vi "WaitForRPM.vi"(7 "Notifier Data":T2, 8 "error in (no error)":errorcluster, 9 "RPM target":dbl, 10 "Data Cluster":T1, 11 "Notifier in":refnum<notifier>) -> (0 "error out":errorcluster, 1 "RPM Target Reached":bool, 2 "STOP Button Pressed":bool, 3 "RPM Timeout":bool, 5 "RPM":dbl)   [LabVIEW 2026, in "Acquisition.lvlib"]
uses:
  Acquisition.lvlib
  controls/NotifierAndDataQueue.ctl
  controls/WaveformChartData.ctl
  Hardware Configuration.ctl
  Settings/Settings.lvlib
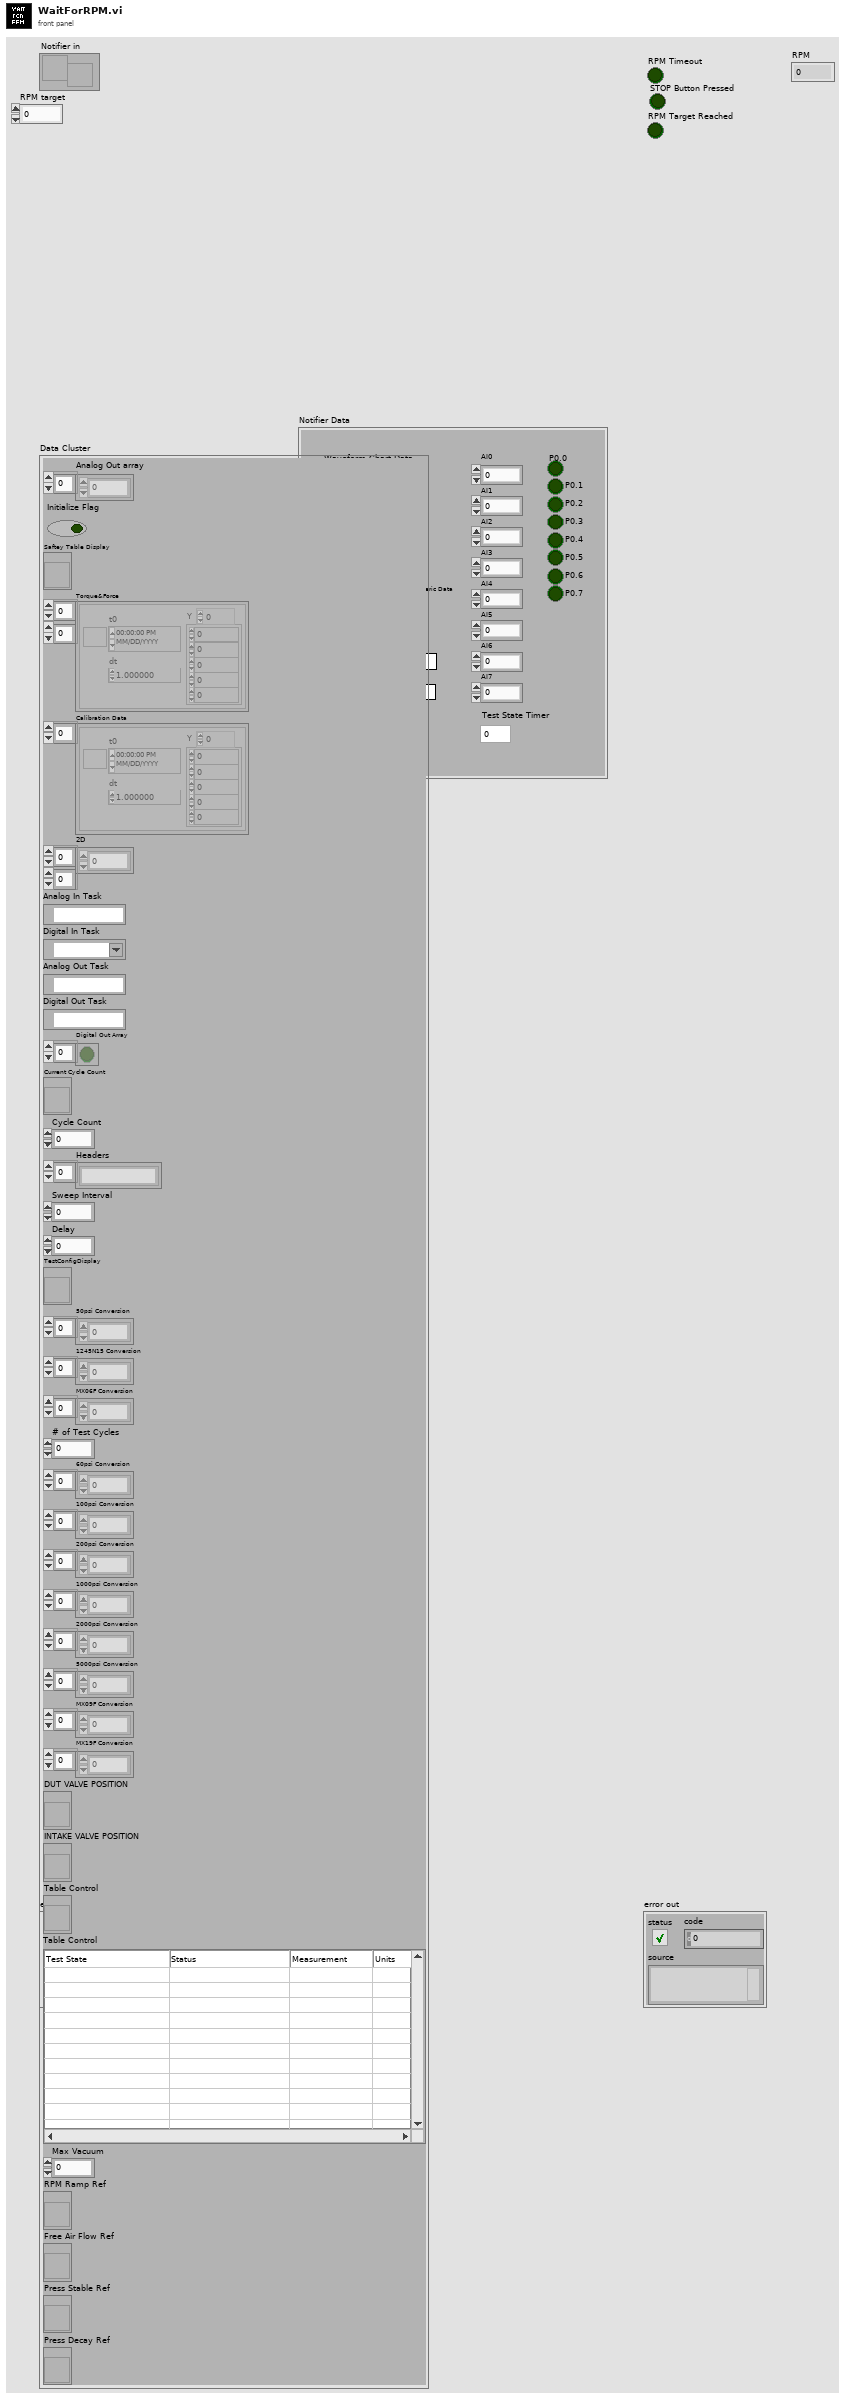
[diagram p1: front panel]
types:
  T1 = typedef "Acquisition.lvlib/Hardware Configuration.ctl" = cluster{"Analog Out array":dbl[], "Initialize Flag":bool, "Saftey Table Display":refnum<vi>, "Torque&Force":waveform(dbl)[][], "Calibration Data":waveform(dbl)[], "2D":dbl[][], "Analog In Task":refnum<k21>, "Digital In Task":refnum<k21>, "Analog Out Task":refnum<k21>, "Digital Out Task":refnum<k21>, "Digital Out Array":bool[], "Current Cycle Count":refnum<vi>, "Cycle Count":u64, "Headers":string[], "Sweep Interval":u64, "Delay":u64, "TestConfigDisplay":refnum<vi>, "50psi Conversion":dbl[], "1245N15 Conversion":dbl[], "MX06F Conversion":dbl[], "# of Test Cycles":u64, "60psi Conversion":dbl[], "100psi Conversion":dbl[], "200psi Conversion":dbl[], "1000psi Conversion":dbl[], "2000psi Conversion":dbl[], "5000psi Conversion":dbl[], "MX09F Conversion":dbl[], "MX19F Conversion":dbl[], "DUT VALVE POSITION":refnum<vi>, "INTAKE VALVE POSITION":refnum<vi>, "Table Control":refnum<vi>, "Table Control":string[][], "Max Vacuum":dbl, "RPM Ramp Ref":refnum<vi>, "Free Air Flow Ref":refnum<vi>, "Press Stable Ref":refnum<vi>, "Press Decay Ref":refnum<vi>}
  T2 = typedef "NotifierAndDataQueue.ctl" = cluster{"Ai0":dbl, "Ai1":dbl, "Ai2":dbl, "Ai3":dbl, "Ai4":dbl, "Ai5":dbl, "Ai6":dbl, "Ai7":dbl, "P0.0":bool, "P0.1":bool, "P0.2":bool, "P0.3":bool, "P0.4":bool, "P0.5":bool, "P0.6":bool, "P0.7":bool, "2D Numeric Data":dbl[][], "String 2":string, "String 1":string, "Waveform Chart Data":T3, "Test State Timer":dbl}
  T3 = typedef "Settings.lvlib/WaveformChartData.ctl" = cluster{"DUT Vacuum":dbl, "Motor RPM":dbl, "DUT RPM":dbl, "Tank Vacuum":dbl}
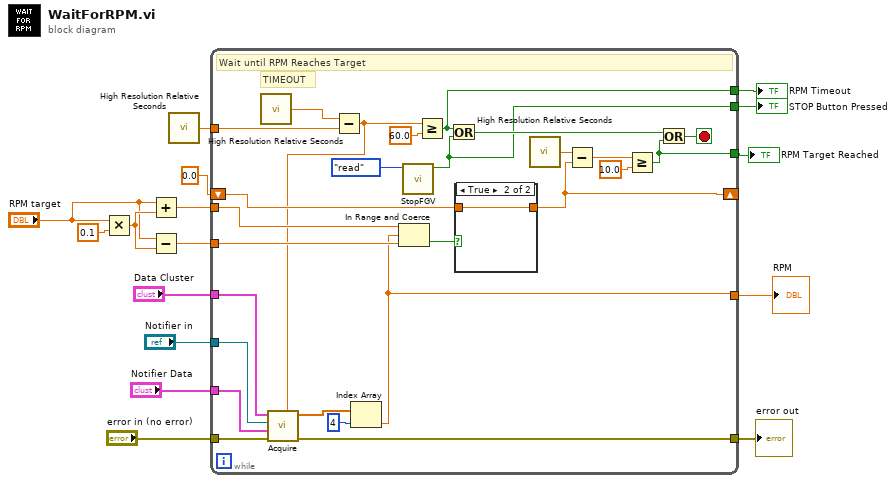
[diagram p0: block diagram]
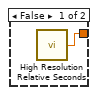
[diagram p2: hidden frame]
diagram:
  n1 = Multiply(x="RPM target", y=0.1) -> (x*y=w8:dbl)
  n2 = Add(x="RPM target", y=w8) -> (x+y=w7:dbl)
  n3 = Subtract(x="RPM target", y=w8) -> (x-y=w6:dbl)
  n4 = call <vilib>:"High Resolution Relative Seconds.vi"() -> ("relative seconds"=w16:dbl)
  n5 = while {
    tunnel: "Notifier in" -> [w40]
    tunnel: "error in (no error)" -> [w42]
    tunnel: [w41] -> w11
    tunnel: "Notifier Data" -> [w37]
    tunnel: "Data Cluster" -> [w36]
    tunnel: w7 -> [w33]
    tunnel: w6 -> [w32]
    shift-right: [w29] -> _
    shift-left: 0.0 ("relative seconds") -> [w28]
    tunnel: w16 -> [w24]
    tunnel: [w21] -> w4
    tunnel: [w20] -> w3
    tunnel: [w19] -> w2
    tunnel: [w18] -> w1
    stop <- w38 stop-if-true
    # "TIMEOUT"
    # "Wait until RPM Reaches Target"
    n6 = call <vilib>:"High Resolution Relative Seconds.vi"() -> ("relative seconds"=w25:dbl)
    n7 = Subtract(x=w25, y=w24) -> (x-y=w17:dbl)
    n8 = call "Acquire.vi"("Test State Timer"=w17, "error in (no error)"=w42, "Notifiier Data"=w37, "notifier out"=w40, "Hardware Resources in"=w36) -> ("error out"=w41:errorcluster, "Averaged Data Array"=w35:dbl[])  [unwired: 4 in, 1 out]
    n9 = Index Array(array=w35, index=4) -> (element=w18:dbl)
    n10 = In Range and Coerce(upper limit=w33, x=w18, lower limit=w32) -> (In Range?=w31:bool)  [unwired: 1 out]
    n11 = call "StopFGV.vi"("Enum"=enum16{"init", "write", "read"}."read") -> ("STOP Out"=w20:bool)  [unwired: 9 in, 1 out]
    n12 = Greater Or Equal?(x=w17, y=60.0) -> (x >= y?=w21:bool)
    n13 = Or(x=w21, y=w20) -> (x .or. y?=w22:bool)
    n14 = case shown="True" w31 {
      tunnel: [w43 w44] -> w29
      tunnel: w28 -> [_ w44]
      frame False {
        n15 = call <vilib>:"High Resolution Relative Seconds.vi"() -> ("relative seconds"=w43:dbl)
      }
      frame True {
      }
    }
    n16 = call <vilib>:"High Resolution Relative Seconds.vi"() -> ("relative seconds"=w30:dbl)
    n17 = Subtract(x=w30, y=w29) -> (x-y=w27:dbl)
    n18 = Greater Or Equal?(x=w27, y=10.0) -> (x >= y?=w19:bool)
    n19 = Or(x=w22, y=w19) -> (x .or. y?=w38:bool)
  }
  "error out" <- w11
  "RPM Timeout" <- w4
  "STOP Button Pressed" <- w3
  "RPM Target Reached" <- w2
  "RPM" <- w1
